vi "Set Calling VI Wnd Topmost & Active.vi"(8 "Error In":errorcluster) -> (0 "Error Out":errorcluster)   [LabVIEW 2021]
doc: "Sets the Caller VIs front panel Topmost (no other windows can be in front), Active (title bar is selected), and gives Focus (keystrokes are directed to the panel).\n\nhttp://lavag.org/topic/12751-how-do-you-make-your-application-window-frontmost/#entry76322\n\nCopyright © 2010 Blue Ridge Test, Inc.\nwww.BlueRidgeTest.com"
uses:
  Windows/System32/user32.dll
panel:
  out "Show\\Rest":i32
  out "Minimized?":i32
  out "FG hWnd":i32
  out "FG ProcID":i32
  out "hWnd ProcID":i32
  out "SetFG\\Attach":i32
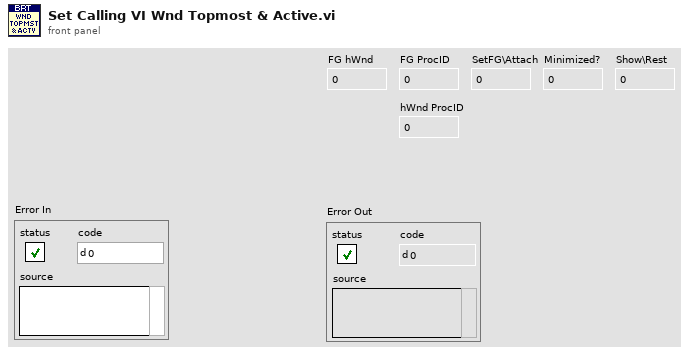
[diagram p1: front panel]
types:
  T1 = enum32{"Invalid", "Standard", "Closed", "Hidden", "Minimized", "Maximized"}
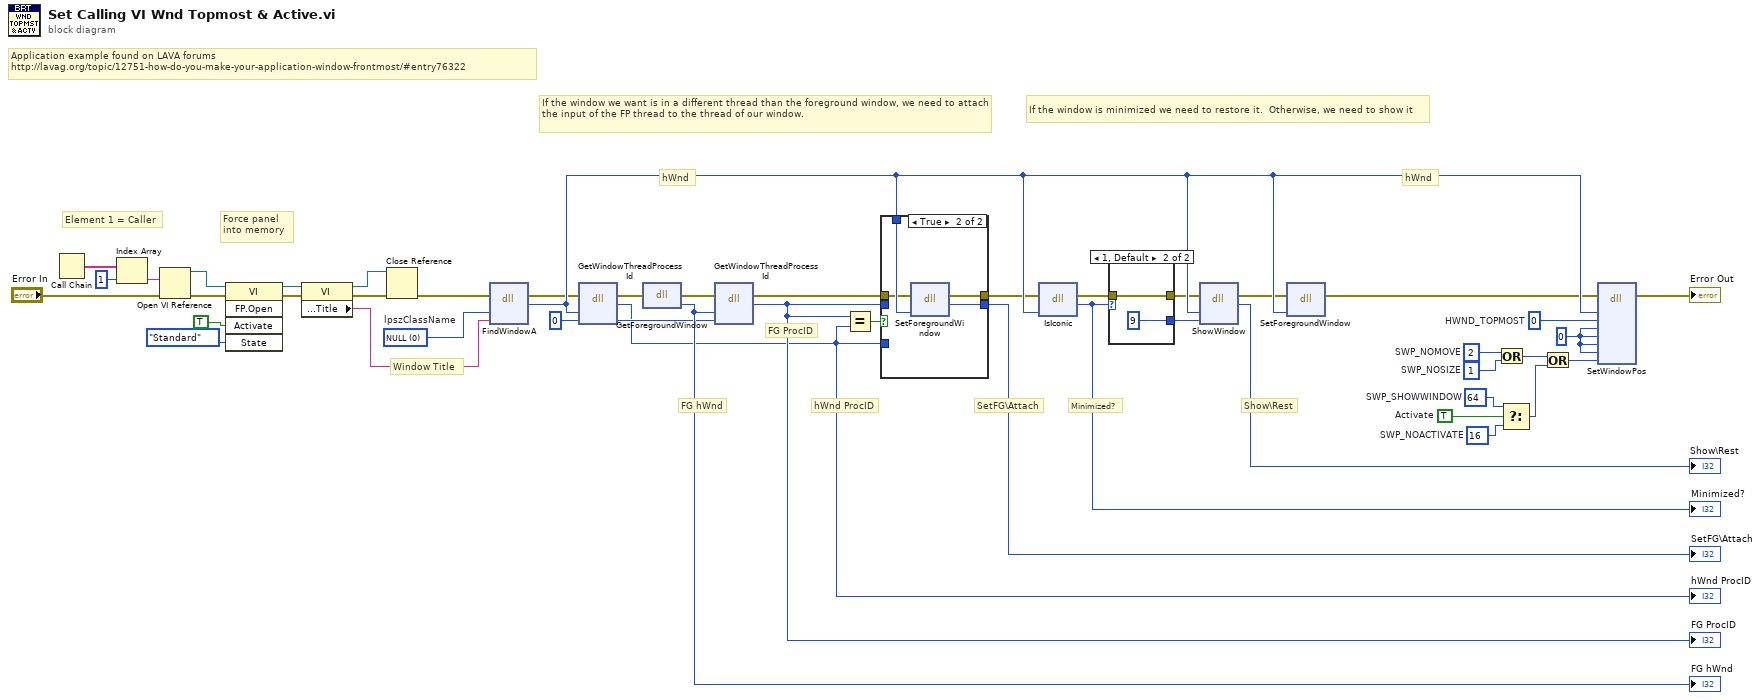
[diagram p0: block diagram]
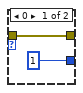
[diagram p2: hidden frame]
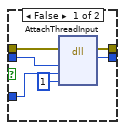
[diagram p3: hidden frame]
diagram:
  w3 = TRUE  # Activate
  w2 = u32 16  # SWP_NOACTIVATE
  w1 = u32 64  # SWP_SHOWWINDOW
  w16 = 0 ("lpdwProcessID")
  w23 = 0  # HWND_TOPMOST
  w28 = u32 2  # SWP_NOMOVE
  w27 = u32 1  # SWP_NOSIZE
  w29 = 0
  w43 = 0 items=["NULL"]  # lpszClassName
  # "Application example found on LAVA forums\nhttp://lavag.org/topic/12751-how-do-you-make-your-application-window-frontmost/#entry76322"
  # "hWnd ProcID"
  # "Show\\Rest"
  # "Minimized?"
  # "SetFG\\Attach"
  # "Force panel\ninto memory"
  # "FG hWnd"
  # "FG ProcID"
  # "hWnd"
  # "If the window is minimized we need to restore it.  Otherwise, we need to show it"
  # "hWnd"
  # "If the window we want is in a different thread than the foreground window, we need to attach the input of the FP thread to the thread of our window."
  # "Window Title"
  # "Element 1 = Caller"
  n1 = Call Chain() -> (call chain=w41:string[])
  n2 = Index Array(array=w41, index=1) -> (element=w40:string)
  n3 = Open VI Reference(vi path=w40, error in (no error)="Error In") -> (vi reference=w37:refnum<vi>, error out=w38:errorcluster)  [unwired: 4 in]
  n4 = invoke class="VI" method="FP.Open"(reference=w37, error in=w38, "Activate"=TRUE ("Activate?"), "State"=T1."Standard") -> (reference out=w35:refnum<vi>, error out=w36:errorcluster)  [unwired: 1 in, 3 out]
  n5 = property class="VI"(reference=w35, error in=w36) -> (reference out=w33:refnum<vi>, error out=w32:errorcluster, "Front Panel.Title"=w34:string)
  n6 = Close Reference(reference=w33, error in (no error)=w32) -> (error out=w31:errorcluster)
  n7 = dll-call lib="C:/Windows/System32/USER32.DLL" fn="FindWindowA" label="FindWindow"(error in=w31, "lpszClassName"=w43, "lpszWindowName"=w34) -> (error out=w19:errorcluster, "hWnd"=w22:u32)  [unwired: 4 in, 1 out]
  n8 = dll-call lib="user32" fn="GetWindowThreadProcessId" label="Get\nWindow\nThread\nProcess\nId"(error in=w19, "hWnd"=w22, "lpdwProcessID"=w16) -> (error out=w11:errorcluster, w10:i32)  [unwired: 4 in, 1 out]
  "hWnd ProcID" <- w10
  n9 = dll-call lib="user32" fn="GetForegroundWindow" label="Get\nForeground\nWindow"(error in=w11) -> (error out=w12:errorcluster, "hWnd"=w17:i32)  [unwired: 2 in, 1 out]
  "FG hWnd" <- w17
  n10 = dll-call lib="user32" fn="GetWindowThreadProcessId" label="Get\nWindow\nThread\nProcess\nId"(error in=w12, "hWnd"=w17, "lpdwProcessID"=w16) -> (error out=w9:errorcluster, w14:i32)  [unwired: 4 in, 1 out]
  "FG ProcID" <- w14
  n11 = Equal?(x=w14, y=w10) -> (x = y?=w15:bool)
  n12 = case shown="True" w15 {
    tunnel: w14 -> [w51 _]
    tunnel: w10 -> [w50 _]
    tunnel: w22 -> [_ w55]
    tunnel: [w48 w54] -> w13
    tunnel: w9 -> [w47 w53]
    tunnel: [w46 w52] -> w21
    frame False {
      n13 = dll-call lib="user32" fn="AttachThreadInput" label="Attach\nThread\nInput"(error in=w47, "idAttach"=w51, "idAttachTo"=w50, "fAttach"=1) -> (error out=w46:errorcluster, w48:i32)  [unwired: 5 in, 1 out]
    }
    frame True {
      n14 = dll-call lib="user32" fn="SetForegroundWindow" label="Set\nForeground\nWindow"(error in=w53, "hWnd"=w55) -> (error out=w52:errorcluster, w54:i32)  [unwired: 3 in, 1 out]
    }
  }
  "SetFG\\Attach" <- w13
  n15 = dll-call lib="user32" fn="IsIconic"(error in=w21, "hWnd"=w22) -> (error out=w4:errorcluster, w8:i32)  [unwired: 3 in, 1 out]
  "Minimized?" <- w8
  n16 = case shown="1, Default" w8 {
    tunnel: [i16 1 ("nCmdshow") i16 9 ("nCmdshow")] -> w7
    tunnel: [w56 w58] -> w5
    tunnel: w4 -> [w56 w58]
    frame 0 {
    }
    frame 1, Default {
    }
  }
  n17 = dll-call lib="C:/Windows/System32/user32.dll" fn="ShowWindow"(error in=w5, "hWnd"=w22, "nCmdshow"=w7) -> (error out=w20:errorcluster, →"Show\\Rest":i32)  [unwired: 4 in, 1 out]
  n18 = dll-call lib="user32" fn="SetForegroundWindow" label="Set\nForeground\nWindow"(error in=w20, "hWnd"=w22) -> (error out=w18:errorcluster)  [unwired: 4 in, 1 out]
  n19 = Or(x=w28, y=w27) -> (x .or. y?=w25:u32)
  n20 = Select(t=w1, s=w3, f=w2) -> (s? t:f=w26:u32)
  n21 = Or(x=w25, y=w26) -> (x .or. y?=w24:u32)
  n22 = dll-call lib="C:/Windows/System32/USER32.DLL" fn="SetWindowPos"(error in=w18, "hWnd"=w22, "hWndInsertAfter"=w23, "left"=w29, "top"=w29, "width"=w29, "height"=w29, "fuFlags"=w24) -> (error out=→"Error Out":errorcluster)  [unwired: 8 in, 3 out]
